vi "Lectura del Com.vi"(8 "error in (no error)":errorcluster, 11 "VISA Refnum in":refnum<visa-resource-name>) -> (0 "error out":errorcluster, 2 "Serial Response":string, 3 "VISA resource name out":refnum<visa-resource-name>)   [LabVIEW 2019, in "Serial Devices.lvlib"]
uses:
  Serial Devices.lvlib
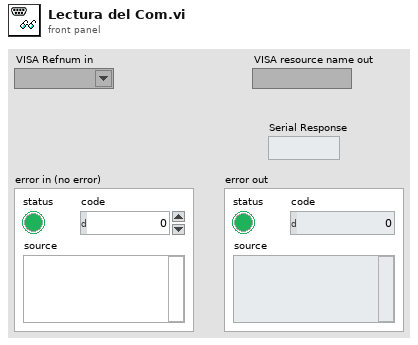
[diagram p1: front panel]
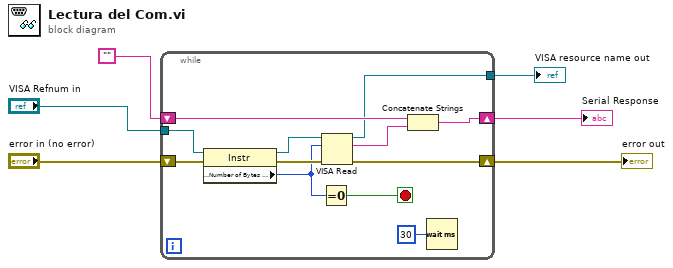
[diagram p0: block diagram]
diagram:
  n1 = while {
    tunnel: "VISA Refnum in" -> [w18]
    shift-right: [w17] -> w5
    shift-left: "error in (no error)" -> [w16]
    shift-right: [w11] -> w2
    shift-left: "" -> [w12]
    tunnel: [w7] -> w1
    stop <- w8 stop-if-true
    n2 = property class="Instr"(reference=w18, error in=w16) -> (reference out=w14:refnum<visa-resource-name>, error out=w15:errorcluster, "Serial Settings:Number of Bytes at Serial Port"=w9:u32)
    n3 = Equal To 0?(x=w9) -> (x = 0?=w8:bool)
    n4 = VISA Read(VISA resource name=w14, byte count=w9, error in (no error)=w15) -> (VISA resource name out=w7:refnum<visa-resource-name>, read buffer=w13:string, error out=w17:errorcluster)  [unwired: 1 out]
    n5 = Concatenate Strings(w12, w13) -> (w11:string)
    n6 = Wait (ms)(milliseconds to wait=u32 30) -> ()  [unwired: 1 out]
  }
  "error out" <- w5
  "Serial Response" <- w2
  "VISA resource name out" <- w1
